vi "test code emballage_ZEBRA_TCPIP.vi"() -> ()   [LabVIEW 2020]
panel:
  in  "Choix imprimante":T1(ring)=enum."Zebra_Medic_1"
  in  "entrйe d'erreur":errorcluster
  out "sortie d'erreur 2":errorcluster caption="sortie d'erreur"
  out "sortie d'erreur":errorcluster
  out "Nom de ressource VISA en sortie":refnum<visa-resource-name>="TLP3844-Z"
  in  "chaine a ecrire":string="^XA\n^KL3\n^SC9600,8,N,1,,N\n^PRA\n^LL1428\n^ML1500\n^MMC\n^LH100,90\r\r^AFB,1,1^FT0,940^FDDestinataire :^FS\n^A0B,34,34^FT0,700^FD EMS Electro Medical System^FS\r\n^AFB,1,1^FT40,940^FDN§ commande : CF-08-0253/2^FS\r^AFB,1,1^FT80,940^FDQuantit‚ : 50/100^FS\r^AFB,1,1^FT120,940^FDVotre r‚f. : EL-360^FS\r^AFB,1,1^FT200,940^FDN§ valves :^FS\r^AFB,1,1^FT235,905^FD(P/N)^FS\r\r^FT588,30\n^BY2,2.0\n^BCI,80,N,N,N\n^FDEL-360 03 08010801 50^FS\r^A0I,30,30^FT441,0^FDEL-360 03 08010801 50^FS\r\r^A0B,24,24^FT200,750^FD  08010001,  08010002,  08010003,  08010004,  08010005^FS\r^A0B,24,24^FT225,750^FD  08010006,  08010007,  08010008,  08010009,  08010010^FS\r^A0B,24,24^FT250,750^FD  08010011,  08010012,  08010013,  08010014,  08010015^FS\r^A0B,24,24^FT275,750^FD  08010016,  08010017,  08010018,  08010019,  08010020^FS\r^A0B,24,24^FT300,750^FD  08010021,  08010022,  08010023,  08010024,  08010025^FS\r^A0B,24,24^FT325,750^FD  08010026,  08010027,  08010028,  08010029,  08010030^FS\r^A0B,24,24^FT350,750^FD  08010031,  08010032,  08010033,  08010034,  08010035^FS\r^A0B,24,24^FT375,750^FD  08010036,  08010037,  08010038,  08010039,  08010040^FS\r^A0B,24,24^FT400,750^FD  08010041,  08010042,  08010043,  08010044,  08010045^FS\r^A0B,24,24^FT425,750^FD  08010046,  08010047,  08010048,  08010049,  08010050^FS\r\r^FT465,940\n^GB0,800,3^FS\n\n^FT650,940\n^BXB,6,0\n^FD12-216C-04521 EQIFIL 417mA 14.4ohm;03838/08-01.07.01;1/2^FS\r^AFB,1,1^FT525,760^FDN§ article FAS :^FS\r^A0B,34,34^FT565,760^FD12-216C-04521 EQIFIL 417mA 14.4ohm^FS\r^AFB,1,1^FT605,760^FDN§ commande FAS :^FS\r^A0B,34,34^FT645,760^FD03838/08-01.07.01^FS\r^AFB,1,1^FT685,760^FDCarton : ^FS\r^A0B,34,34^FT685,616^FD1/2^FS\r\r^PQ1\n^XZ\r"
  # "Grande etiquette - 1 code bar 2D + scan"
  # "Grande etiquette - 1 code bar 2D"
  # "ZB\nUS\nq592\nD7\nN\nR166,48\nI8,12,001\nA504,828,2,1,1,1,N,\"FASmedic s.a.\"\nA504,812,2,1,1,1,N,\"Zone industrielle\"\nA504,796,2,1,1,1,N,\"CH-1607 Pal‚zieux-Gare\"\nA504,780,2,1,1,1,N,\"T‚l.+41(0)21 907 79 71\"\nA504,764,2,1,1,1,N,\"www.fasmedic.com\"\nA34,712,3,2,1,1,N,\"Destinataire:EMS Electro Medical System\"\nA74,712,3,2,1,1,N,\"Nшcommande:CF-08-0253/2\"\nA114,712,3,2,1,1,N,\"Carton:1/2\"\nA154,712,3,2,1,1,N,\"Quantit‚:50/100\"\nA194,712,3,2,1,1,N,\"Votre ref.:EL-360\"\nLO258,112,2,600\nb404,112,D,4,\"12-216C-04521 EQIFIL 417mA 14.4ohm     03838/08-07.01.01\"\nA318,712,3,2,1,1,N,\"Nшarticle FAS:\"\nA358,712,3,3,1,1,N,\"12-216C-04521 EQIFIL 417mA 14.4ohm\"\nA398,712,3,2,1,1,N,\"Nшcommande FAS:\"\nA438,712,3,3,1,1,N,\"03838/08-07.01.01\"\nB318,64,2,3,1,2,56,N,\"EL-360 03 08010801\"\nA318,0,2,3,1,1,N,\"EL-360 03 08010801\"\nGW265,824,32,61,яяяяяяяяяяяяяяяяяяяяяяяяяяяяяяяЏяяяяяяяяяяяяяяяяяяяяяяяяяяяяяяюяяяяяяяяяяяяяяяяяяяяяяяяяяяяяяшяяяяяяяяяяяяяяяяяяяяяяяяяяяяяяАяяяяяяяяяяяяяяяяяяяяяяяяяяяяяяяяяяяяяяяяяяяяяяяяяяяяяяяяяяяяяяяяяяяяяяяяяяяяяяяяяяяяяяяяяюяяяяяяяяяяяяяяяяяяяяяяяяяяяяяюяяяяяяяяяяяяяяяяяяяяяяяяяяяяяюяяяяяяяяяяяяяяяяяяяяяяяяяяяяяьяяяяяяяяяяяяяяяяяяяяяяяяяяяяяьяяяяяяяяяяяяяяяяяяяяяяяяяяяяяшяЃяяяяьяяяяяяаяяяЂ?яяяяяяяшюП<ярьящяуя?Аяю8ш>П0x?БрьящяуьАяь0щяЏП#яЏь|ящяушАяшpуяЗП'яЏю<ящяурАяр`гягПяЏ?яящяуарАшяаазяуПяЗ?яњящяуашАьяЂАЗяуПяж?яњящяуашАьяАПяыПяжяЬящяуаяяАья~АяящПязяяМящяуаяяАшяЂяящП?язяяМящяуаяАаяЂяящП?ячяяМящяур?АяЂ?яящП?яцящяурАяА?яящП?яцящяушАяаяящП?яжяМящяуяАяряящПяжяЬящяуярАяяряяыПяжяњящягяяаАяяяшяПяуПяж?яњящягррАяяяяяяяяяяЗяуПяЗ?яясягррАшяяяяяяязягПяП?я>ясягрраряЂягязП'яЏџю>аяГраяЂ0ясяЏП#я‡ь~?А“шря0яшяП1ь?ГряЊ3ьшюpяь?П8аяЂsьью`яяЃяя?ѓяюяаяГяяАяяАяяьаяяяяя?яяяяяяяяяяяяяяяяяяьАяяяяя?яяяяяяяяяяяяяяяяяюьАяяяяя?яяяяяяяяяяяяяяяяяюшАяяяяя?яяяяяяяяяяяяяяяяяьшЂяяяяП?яяяяяяяяяяяяяяяяярЂяяяяП?яяяяяяяяяяяяяяяяяяр?яяяяП?яяяяяяяяяяяяяяяяяяр?яяяяП?яяяяяяяяяяяяяяяяяяаяяяяП?яяяяяяяяяяяяяяяяяяаяяяяяяяяяяяяяяяяяяяяяяяяАяяяяяяяяяяяяяяяяяяяяяяяяяяяАяяяяяяяяяяяяяяяяяяяяяяяяяяяЂяяяяяяяяяяяяяяяяяяяяяяяяяяяяяЂяяяяяяяяяяяяяяяяяяяяяяяяяяяяяЂ?яяяяяяяяяяяяяяяяяяяяяяяяяяяяяЂ?яяяяяяяяяяяяяяяяяяяяяяяяяяяяяЂ?яяяяяяяяяяяяяяяяяяяяяяяяяяяяяЂяяяяяяяяяяяяяяяяяяяяяяяяяяяяяАяяяяяяяяяяяяяяяяяяяяяяяяяяяяяаяяяяяяяяяяяяяяяяяяяяяяяяяяяяяяаяяяяяяяяяяяяяяяяяяяяяяяяяяяяяяряяяяяяяяяяяяяяяяяяяяяяяяяяяяяяр?яяяяяяяяяяяяяяяяяяяяяяяяяяяяяяшяяяяяяяяяяяяяяяяяяяяяяяяяяяяяящяяяяяя\nP1"
  # "FAS Medic RETOUR"
  # "FAS Medic normal"
  # "^XA\n^KL3\n^SC9600,8,N,1,,N\n^PRA\n^LL1428\n^ML888\n^MMC\n^LH100,90\n\n^AFB,1,1^FT0,940^FDCustomer : EMS Electro Medical System^FS\n^AFB,1,1^FT40,940^FDOrder Nb. : CF-08-0253/2^FS\n^AFB,1,1^FT80,940^FDQuantity : 25/25^FS\n^AFB,1,1^FT120,940^FDYour ref. : EL-360^FS\n^AFB,1,1^FT200,940^FDValve Nb. :^FS\n^AFB,1,1^FT235,905^FD(P/N)^FS\n\n^FT588,30\n^BY2,2.0\n^BCI,80,N,N,N\n^FDEL-360 03 08010802 25^FS\n^A0I,30,30^FT441,0^FDEL-360 03 08010802 25^FS\n\n^A0B,24,24^FT200,750^FD  08010001,  08010002,  08010003,  08010004^FS\n^A0B,24,24^FT225,750^FD  08010005,  08010006,  08010007,  08010008^FS\n^A0B,24,24^FT250,750^FD  08010009,  08010010,  08010011,  08010012^FS\n^A0B,24,24^FT275,750^FD  08010013,  08010014,  08010015,  08010016^FS\n^A0B,24,24^FT300,750^FD  08010017,  08010018,  08010019,  08010020^FS\n^A0B,24,24^FT325,750^FD  08010022,  08010030,  08010099,  08020006^FS\n^A0B,24,24^FT350,750^FD  08020066^FS\n^A0B,24,24^FT375,750^FD  ^FS\n^A0B,24,24^FT400,750^FD  ^FS\n^A0B,24,24^FT425,750^FD  ^FS\n\n^FT465,940\n^GB0,800,3^FS\n\n^FT650,940\n^BXB,6,0\n^FD12-216C-04521 EQIFIL 417mA 14.4ohm;03838/08-01.07.01;1/1^FS\n^AFB,1,1^FT525,760^FDFAS Part Number :^FS\n^A0B,30,30^FT560,760^FD12-216C-04521 EQIFIL 417mA 14.4ohm^FS\n^AFB,1,1^FT595,760^FDFAS Order Nb. :^FS\n^A0B,30,30^FT630,760^FD03838/08-01.07.01^FS\n^AFB,1,1^FT665,760^FDBox : ^FS\n^A0B,30,30^FT665,664^FD1/1^FS\n\n^PQ1\n^XZ"
  # "^XA\n^KL3\n^SC9600,8,N,1,,N\n^PRA\n^LL1428\n^ML888\n^MMC\n^LH100,90\n\n^AFB,1,1^FT0,940^FDCustomer : EMS Electro Medical System^FS\n^AFB,1,1^FT40,940^FDOrder Nb. : CF-08-0253/2^FS\n^AFB,1,1^FT80,940^FDQuantity : 25/25^FS\n^AFB,1,1^FT120,940^FDYour ref. : EL-360^FS\n^AFB,1,1^FT200,940^FDValve Nb. :^FS\n^AFB,1,1^FT235,905^FD(P/N)^FS\n\n^AVI,1,1^FT370,26^FDRETOUR^FS\n\n^A0B,24,24^FT200,750^FD  08010001,  08010002,  08010003,  08010004^FS\n^A0B,24,24^FT225,750^FD  08010005,  08010006,  08010007,  08010008^FS\n^A0B,24,24^FT250,750^FD  08010009,  08010010,  08010011,  08010012^FS\n^A0B,24,24^FT275,750^FD  08010013,  08010014,  08010015,  08010016^FS\n^A0B,24,24^FT300,750^FD  08010017,  08010018,  08010019,  08010020^FS\n^A0B,24,24^FT325,750^FD  08010022,  08010030,  08010099,  08020006^FS\n^A0B,24,24^FT350,750^FD  08020066^FS\n^A0B,24,24^FT375,750^FD  ^FS\n^A0B,24,24^FT400,750^FD  ^FS\n^A0B,24,24^FT425,750^FD  ^FS\n\n^FT465,940\n^GB0,800,3^FS\n\n^FT650,940\n^BXB,6,0\n^FD12-216C-04521 EQIFIL 417mA 14.4ohm;R03838/08-01.07.01;1/1^FS\n^AFB,1,1^FT525,760^FDFAS Part Number :^FS\n^A0B,30,30^FT560,760^FD12-216C-04521 EQIFIL 417mA 14.4ohm^FS\n^AFB,1,1^FT595,760^FDFAS Order Nb. :^FS\n^A0B,30,30^FT630,760^FDR03838/08-01.07.01^FS\n^AFB,1,1^FT665,760^FDBox : ^FS\n^A0B,30,30^FT665,664^FD1/1^FS\n\n^PQ1\n^XZ"
  # "100"
  # "^A0I,30,30^FT485,0^FD MK01852  09 08010802 50^FS"
  # "520"
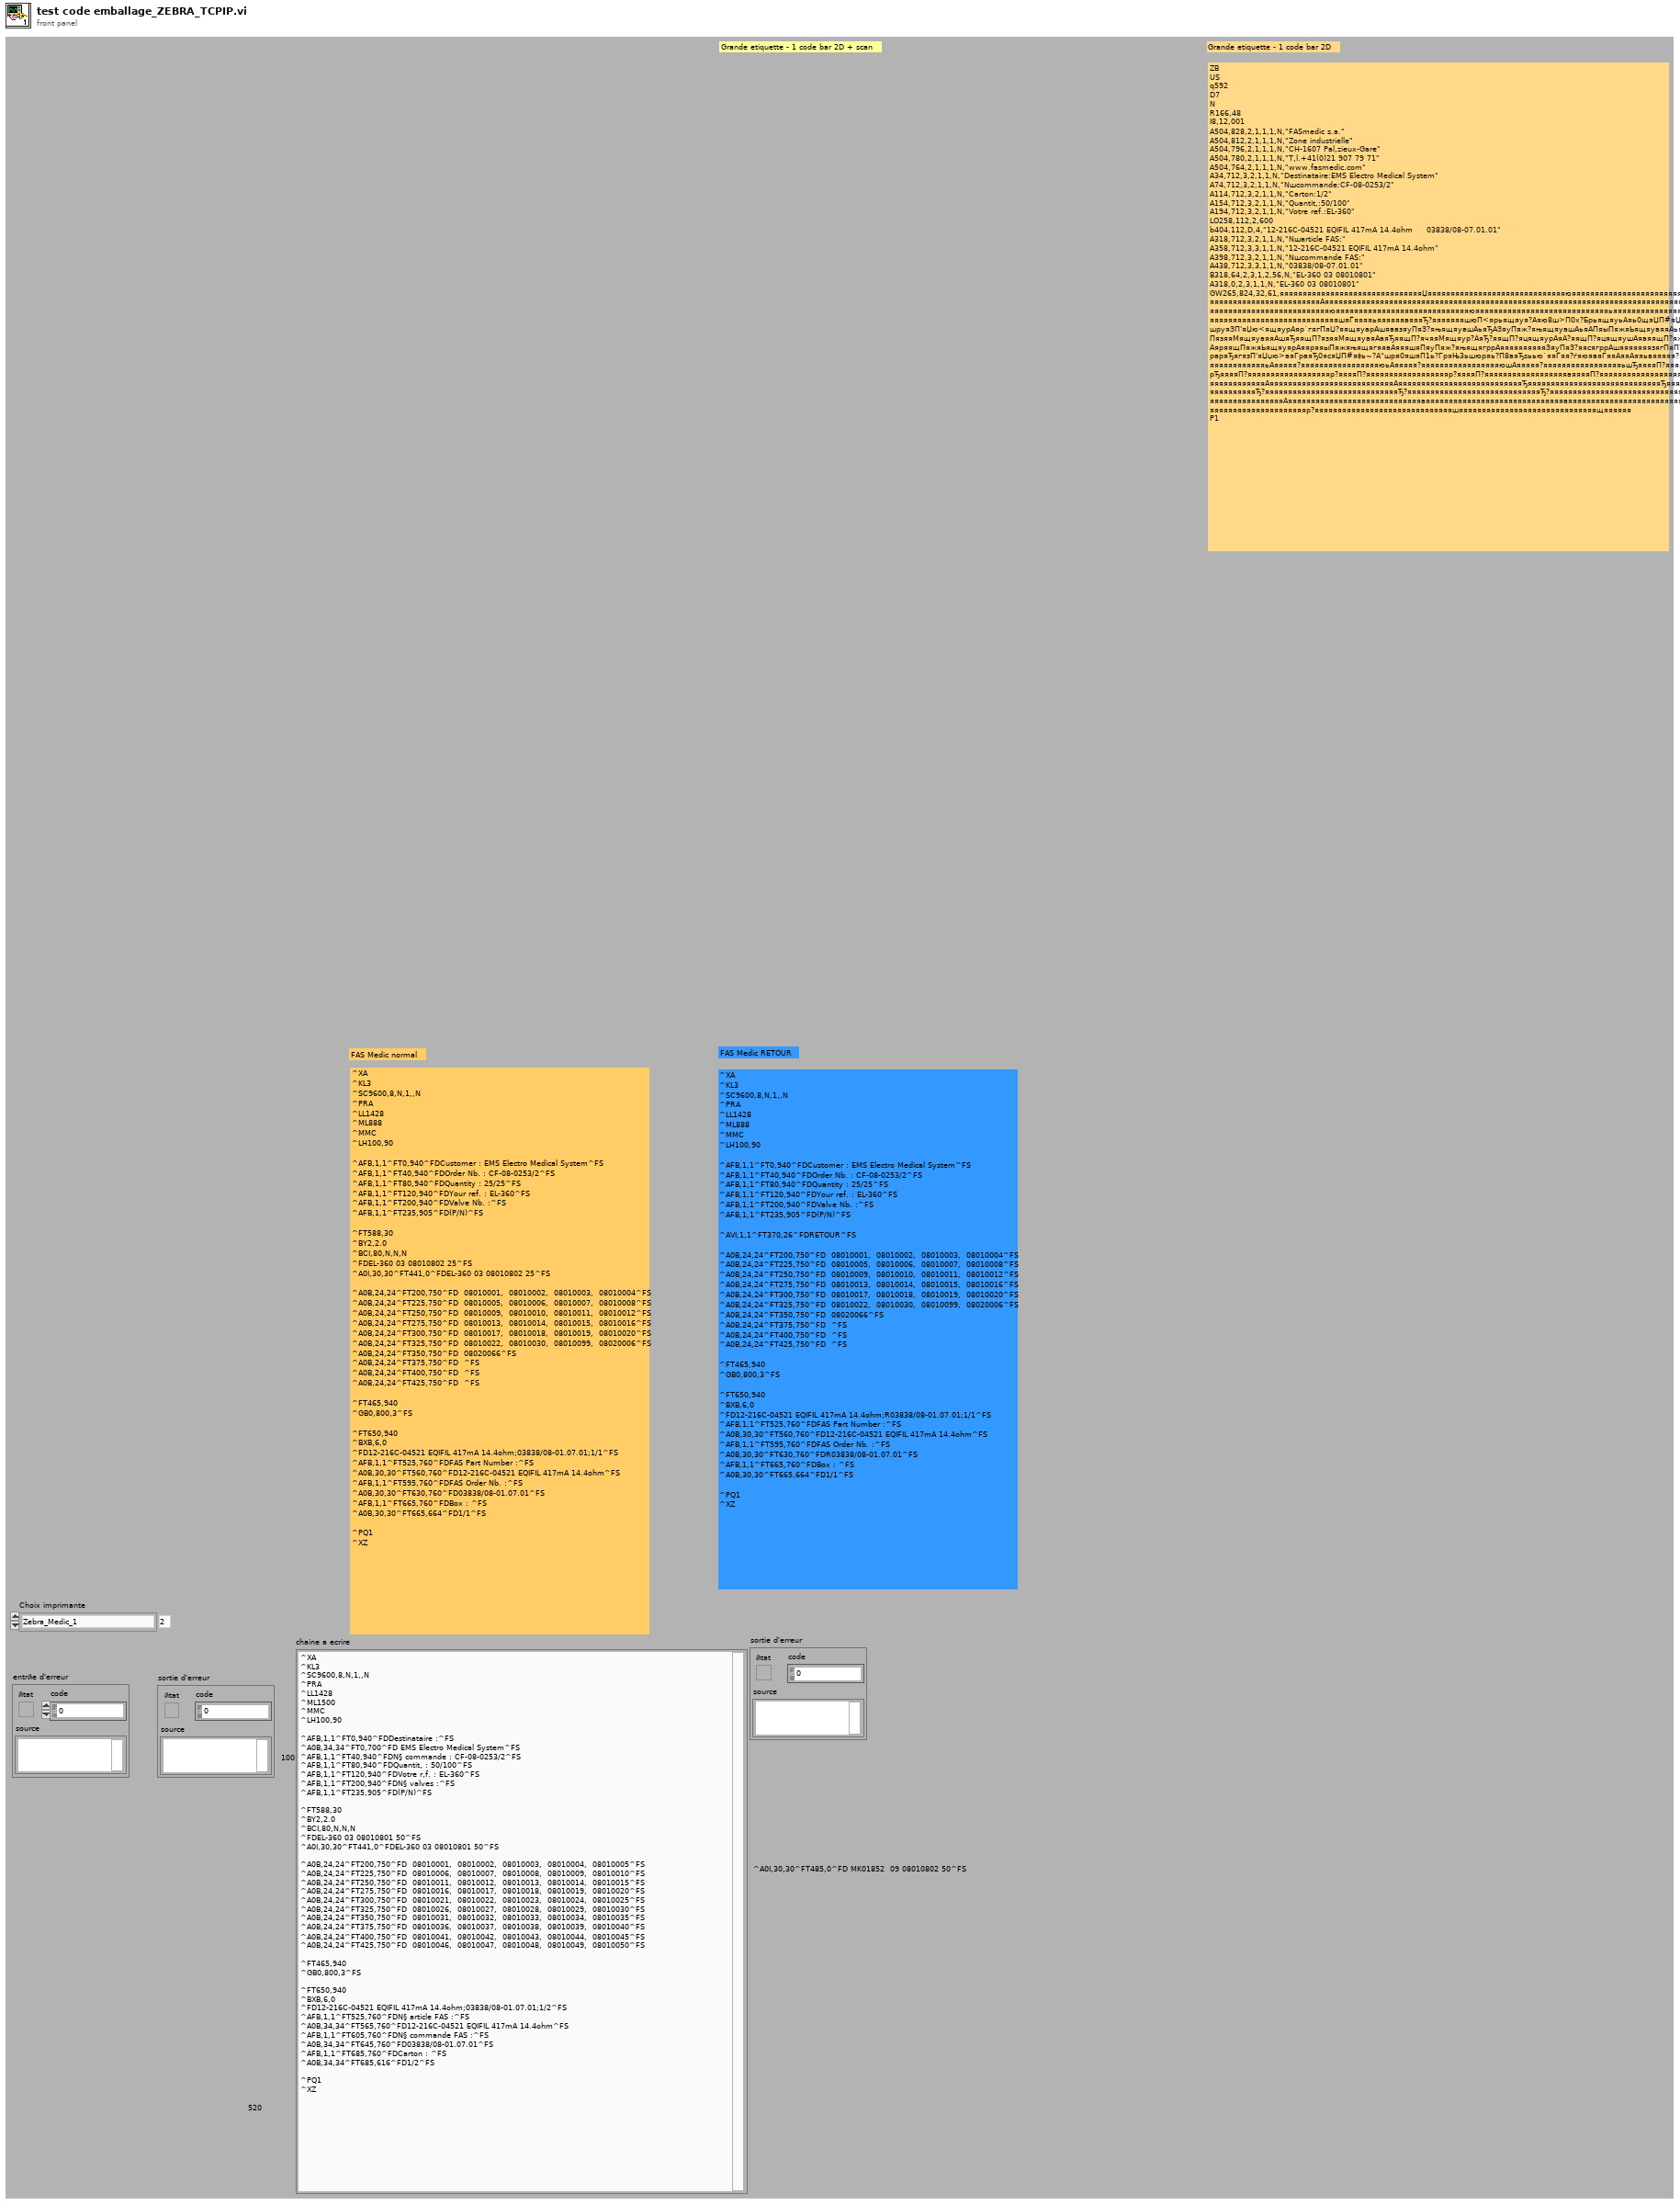
[diagram p1: front panel]
types:
  T1 = enum16{"Zebra_Medic_emballage2", "Zebra_Medic_2", "Zebra_Medic_1", "Zebra_Flat_emballage"}
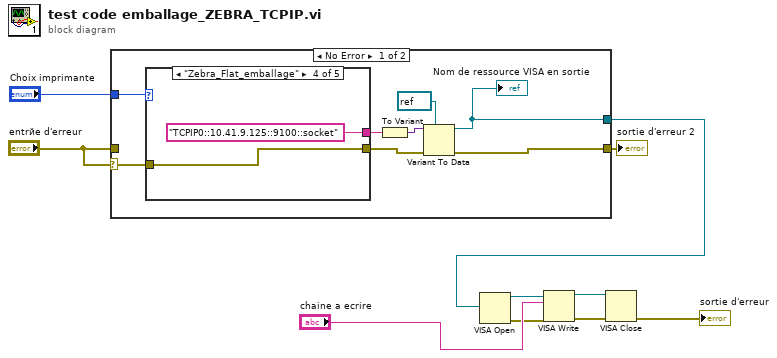
[diagram p0: block diagram]
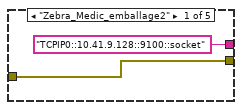
[diagram p2: hidden frame]
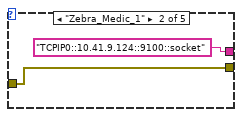
[diagram p3: hidden frame]
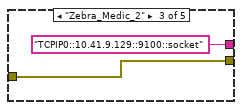
[diagram p4: hidden frame]
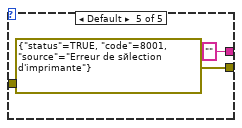
[diagram p5: hidden frame]
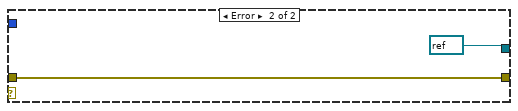
[diagram p6: hidden frame]
diagram:
  n1 = case shown="No Error" "entrйe d'erreur" {
    selector: "entrйe d'erreur" -> [w13 _]
    tunnel: [w15 w30] -> w4
    tunnel: "entrйe d'erreur" -> [_ w30]
    tunnel: "Choix imprimante" -> [w14 _]
    tunnel: [w11 refnum<visa-resource-name> refnum ("Nom de ressource VISA en sortie")] -> w1
    frame No Error {
      n2 = case shown="\"Zebra_Flat_emballage\"" w14 {
        tunnel: ["TCPIP0::10.41.9.128::9100::socket" "TCPIP0::10.41.9.124::9100::socket" "TCPIP0::10.41.9.129::9100::socket" "TCPIP0::10.41.9.125::9100::socket" ""] -> w18
        tunnel: w13 -> [w20 w22 w23 w26 _]
        tunnel: [w20 w22 w23 w26 errorcluster {"status"=TRUE, "code"=8001, "source"="Erreur de sйlection d'imprimante"} ("error IO")] -> w12
        frame "Zebra_Medic_emballage2" {
        }
        frame "Zebra_Medic_1" {
        }
        frame "Zebra_Medic_2" {
        }
        frame "Zebra_Flat_emballage" {
        }
        frame Default {
        }
      }
      n3 = To Variant(anything=w18) -> (Variant=w17:variant)
      n4 = Variant To Data(error in=w12, type=refnum<visa-resource-name> refnum ("Nom de ressource VISA en sortie"), Variant=w17) -> (data=w11:refnum<visa-resource-name>, error out=w15:errorcluster)
      "Nom de ressource VISA en sortie" <- w11
    }
    frame Error {
    }
  }
  "sortie d'erreur 2" <- w4
  n5 = VISA Open(VISA resource name=w1) -> (VISA resource name=w9:refnum<visa-resource-name>, error out=w7:errorcluster)  [unwired: 4 in]
  n6 = VISA Write(VISA resource name=w9, write buffer="chaine a ecrire", error in (no error)=w7) -> (VISA resource name out=w10:refnum<visa-resource-name>, error out=w6:errorcluster)  [unwired: 1 out]
  n7 = VISA Close(VISA resource name=w10, error in (no error)=w6) -> (error out=→"sortie d'erreur":errorcluster)
